vi "Delete Records.vi"(7 "Bulk Delete?":bool, 8 "Error In (no error)":errorcluster, 10 "Expenses Tracker Records In":refnum<class "Expenses Tracker Record.lvclass">[](array[class]), 11 "SQLite DB Operator In":refnum<class "SQLite DB Operator.lvclass">) -> (0 "Error Out":errorcluster, 2 "Expenses Tracker Records Out":refnum<class "Expenses Tracker Record.lvclass">[](array[class]), 3 "SQLite DB Operator Out":refnum<class "SQLite DB Operator.lvclass">)   [LabVIEW 2023, in "SQLite DB Operator.lvclass"]
uses:
  SQLite DB Operator.lvclass
  SQLite DB Operator.lvclass/SQLite DB Operator.ctl
  <vilib>/drjdpowell/SQLite Library/SQL Statement/SQL Statement.lvclass
  <vilib>/drjdpowell/SQLite Library/SQL Connection/Connection.lvclass
  Private/VIs/Prepare Insert Row Command.vi
  Private/VIs/Bind Insert Command Parameters.vi
  Interfaces/Expenses Tracker Record/Expenses Tracker Record.lvclass
  <vilib>/drjdpowell/SQLite Library/Transaction Helpers/Transaction.lvlib
  Private/VIs/Prepare Delete Row Command.vi
  Private/VIs/Bind Delete Command Parameters.vi
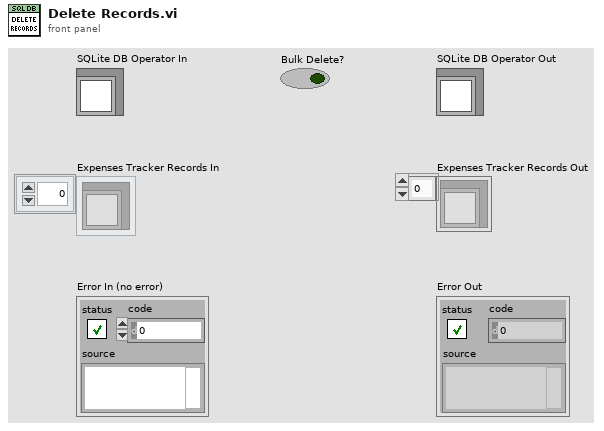
[diagram p1: front panel]
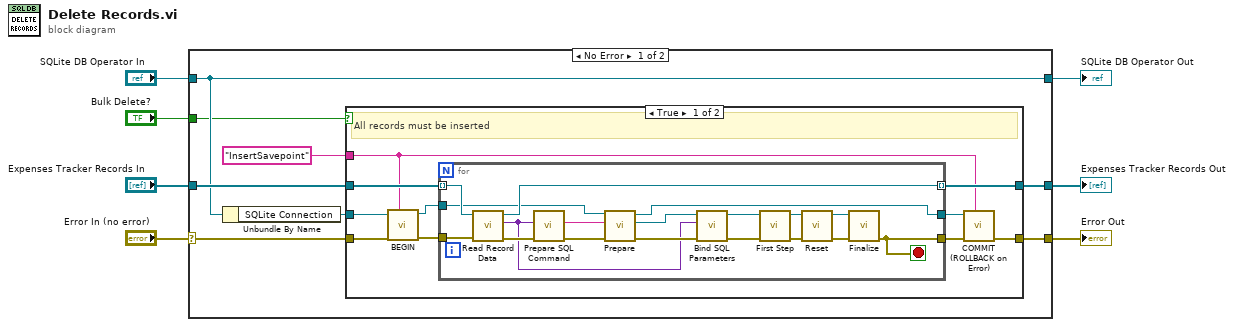
[diagram p0: block diagram]
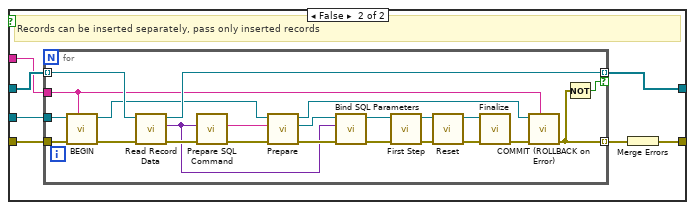
[diagram p2: hidden frame]
diagram:
  n1 = case shown="No Error" "Error In (no error)" {
    selector: "Error In (no error)" -> [w13 w76]
    tunnel: [w11 w76] -> w5
    tunnel: [w14 w75] -> w7
    tunnel: "SQLite DB Operator In" -> [w14 w75]
    tunnel: "Expenses Tracker Records In" -> [w15 w74]
    tunnel: [w10 w74] -> w2
    tunnel: "Bulk Delete?" -> [w8 _]
    frame No Error {
      n2 = Unbundle By Name(w14) -> ("SQLite Connection"=w12:refnum<class "Connection.lvclass">)
      n3 = case shown="True" w8 {
        tunnel: w15 -> [w25 w50]
        tunnel: w13 -> [w22 w49]
        tunnel: w12 -> [w21 w48]
        tunnel: [w16 w44] -> w11
        tunnel: [w24 w46] -> w10
        tunnel: "InsertSavepoint" ("Savepoint name") -> [w23 w45]
        frame True {
          # "All records must be inserted"
          n4 = call <vilib>:"BEGIN.vi"("Savepoint name"=w23, "error in (no error)"=w22, "SQLite Connection in"=w21) -> ("error out"=w20:errorcluster, "SQLite Connection"=w19:refnum<class "Connection.lvclass">)  [unwired: 7 in]
          n5 = for {
            tunnel: w25 -> [w31] mode=indexing
            tunnel: [w30] -> w24 mode=indexing
            tunnel: w20 -> [w29]
            tunnel: w19 -> [w28]
            tunnel: [w26] -> w18
            tunnel: [w27] -> w17
            stop <- w26 stop-if-true
            n6 = call-dynamic "Read Record Data.vi"("Error In (no error)"=w29, "Expenses Tracker Record In"=w31) -> ("Error Out"=w39:errorcluster, "Record"=w33:variant, "Expenses Tracker Record Out"=w30:refnum<class "Expenses Tracker Record.lvclass">)  [unwired: 7 in]
            n7 = call-poly "Prepare SQL Command.vi"("Error In (no error)"=w39, "Record"=w33) -> ("Error Out"=w35:errorcluster, "Insert SQL Command"=w32:string)  [unwired: 8 in]
            n8 = call <vilib>:"Prepare.vi"("error in (no error)"=w35, "SQL"=w32, "SQLite Connection in"=w28) -> ("error out"=w34:errorcluster, "SQL Statement"=w36:refnum<class "SQL Statement.lvclass">, "SQLite Connection"=w27:refnum<class "Connection.lvclass">)  [unwired: 4 in, 2 out]
            n9 = call-poly "Bind SQL Parameters.vi"("Error In (no error)"=w34, "Record"=w33, "SQL Statement In"=w36) -> ("Error Out"=w37:errorcluster, "SQL Statement Out"=w38:refnum<class "SQL Statement.lvclass">)  [unwired: 7 in]
            n10 = call <vilib>:"First Step.vi"("error in (no error)"=w37, "SQL Statement in"=w38) -> ("error out"=w41:errorcluster, "SQL Statement"=w40:refnum<class "SQL Statement.lvclass">)  [unwired: 7 in, 1 out]
            n11 = call <vilib>:"Reset.vi"("error in (no error)"=w41, "SQL Statement in"=w40) -> ("error out"=w43:errorcluster, "SQL Statement"=w42:refnum<class "SQL Statement.lvclass">)  [unwired: 8 in]
            n12 = call <vilib>:"Finalize.vi"("error in (no error)"=w43, "SQL Statement in"=w42) -> ("error out"=w26:errorcluster)  [unwired: 9 in]
          }
          n13 = call <vilib>:"COMMIT (ROLLBACK on Error).vi"("Savepoint name"=w23, "error in (no error)"=w18, "SQLite Connection in"=w17) -> ("error out"=w16:errorcluster)  [unwired: 7 in, 1 out]
        }
        frame False {
          # "Records can be inserted separately, pass only inserted records"
          n14 = for {
            tunnel: w49 -> [w59]
            tunnel: w50 -> [w61] mode=indexing
            tunnel: [w51] -> w47 mode=indexing
            tunnel: [w60] -> w46 mode=indexing if=w54
            tunnel: w45 -> [w55]
            tunnel: w48 -> [w57]
            n15 = call <vilib>:"BEGIN.vi"("Savepoint name"=w55, "error in (no error)"=w59, "SQLite Connection in"=w57) -> ("error out"=w58:errorcluster, "SQLite Connection"=w56:refnum<class "Connection.lvclass">)  [unwired: 7 in]
            n16 = call-dynamic "Read Record Data.vi"("Error In (no error)"=w58, "Expenses Tracker Record In"=w61) -> ("Error Out"=w69:errorcluster, "Record"=w63:variant, "Expenses Tracker Record Out"=w60:refnum<class "Expenses Tracker Record.lvclass">)  [unwired: 7 in]
            n17 = call-poly "Prepare SQL Command.vi"("Error In (no error)"=w69, "Record"=w63) -> ("Error Out"=w65:errorcluster, "Insert SQL Command"=w62:string)  [unwired: 8 in]
            n18 = call <vilib>:"Prepare.vi"("error in (no error)"=w65, "SQL"=w62, "SQLite Connection in"=w56) -> ("error out"=w64:errorcluster, "SQL Statement"=w66:refnum<class "SQL Statement.lvclass">, "SQLite Connection"=w52:refnum<class "Connection.lvclass">)  [unwired: 4 in, 2 out]
            n19 = call-poly "Bind SQL Parameters.vi"("Error In (no error)"=w64, "Record"=w63, "SQL Statement In"=w66) -> ("Error Out"=w67:errorcluster, "SQL Statement Out"=w68:refnum<class "SQL Statement.lvclass">)  [unwired: 7 in]
            n20 = call <vilib>:"First Step.vi"("error in (no error)"=w67, "SQL Statement in"=w68) -> ("error out"=w71:errorcluster, "SQL Statement"=w70:refnum<class "SQL Statement.lvclass">)  [unwired: 7 in, 1 out]
            n21 = call <vilib>:"Reset.vi"("error in (no error)"=w71, "SQL Statement in"=w70) -> ("error out"=w73:errorcluster, "SQL Statement"=w72:refnum<class "SQL Statement.lvclass">)  [unwired: 8 in]
            n22 = call <vilib>:"Finalize.vi"("error in (no error)"=w73, "SQL Statement in"=w72) -> ("error out"=w53:errorcluster)  [unwired: 9 in]
            n23 = call <vilib>:"COMMIT (ROLLBACK on Error).vi"("Savepoint name"=w55, "error in (no error)"=w53, "SQLite Connection in"=w52) -> ("error out"=w51:errorcluster)  [unwired: 7 in, 1 out]
            n24 = Not(x=w51) -> (.not. x?=w54:bool)
          }
          n25 = Merge Errors(w47) -> (w44:errorcluster)
        }
      }
    }
    frame Error {
    }
  }
  "Error Out" <- w5
  "SQLite DB Operator Out" <- w7
  "Expenses Tracker Records Out" <- w2
